vi "Restore Startup Configuration.vi"(8 "error in (no error)":errorcluster, 10 "Startup Configuration File":path=path "C:/Data/Config/start-up.cfg", 11 "Monitor-Pulse in":refnum<class "LabActor.lvclass">) -> (0 "error out":errorcluster, 2 "Startup Configuration":T1={"Load Modules"=[], "External Modules Loaders"=[], "Root Data Folder"=path "C:/Data"}, 3 "Monitor-Pulse out":refnum<class "LabActor.lvclass">)   [LabVIEW 2018, in "LabActor.lvclass"]
uses:
  LabActor.lvclass
  Controllers/Application Controller/Start-up Configuration.ctl
  Controllers/Application Controller/Module Types.ctl
  LabActor.lvclass/LabActor.ctl
  <vilib>/Utility/error.llb/Error Cluster From Error Code.vi
  <vilib>/ErrorRing/Error Ring.xnode
  Controllers/Application Controller/Application Controller.lvclass
  <vilib>/Utility/config.llb/NI_LVConfig.lvlib
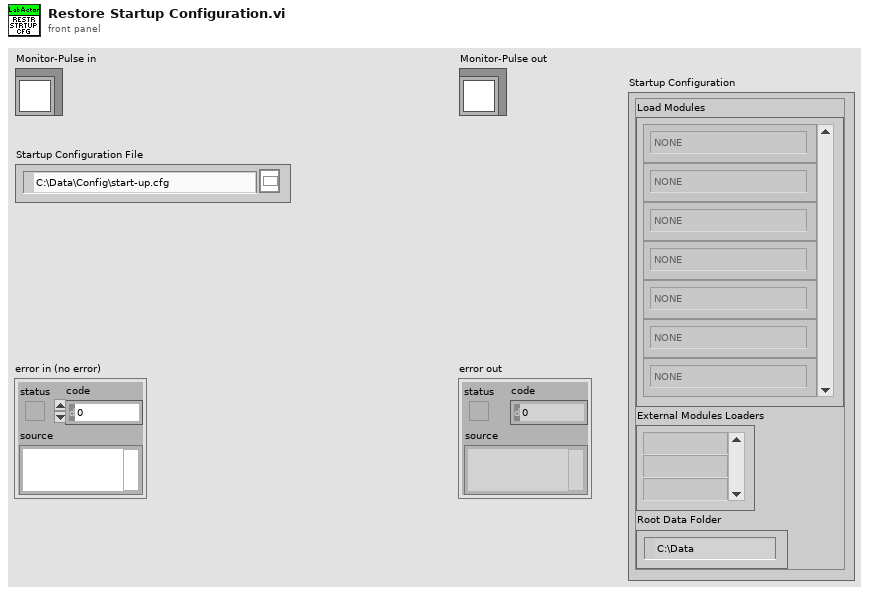
[diagram p1: front panel]
types:
  T1 = typedef "Start-up Configuration.ctl" = cluster{"Load Modules":T2[], "External Modules Loaders":string[], "Root Data Folder":path}
  T2 = typedef "Module Types.ctl" = enum16{"NONE", "NI-DAQmx", "NI-Scope", "Red Pitaya Digitizer", "GaGe", "VISA Device", "Red Pitaya Lockin", "Monitor Controller", "Pulse Controller", "Integrate Pulse", "Lockin Processor", "File converter", "NHMFL Synthesizer", "Micron Hyperion", "Spectrum Recorder", "Resonance Detector", "TCP Communications", "Format Resonances", "Ruby Spectra", "PID Controller"}
  T3 = typedef "NI_LVConfig.lvlib/Config Data RefNum.ctl" = refnum<k1>
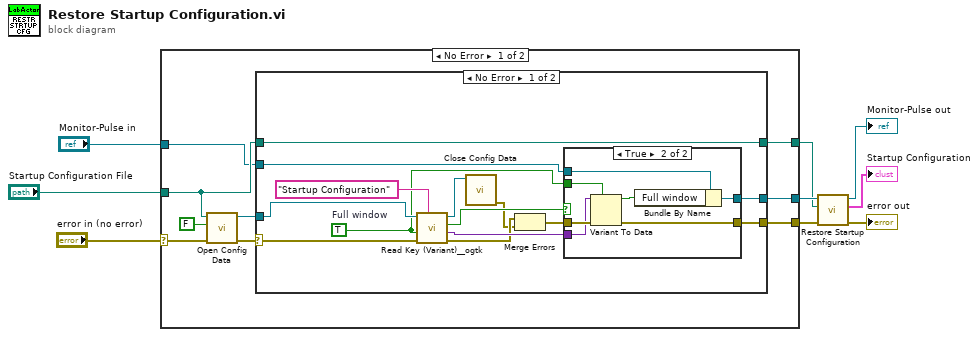
[diagram p0: block diagram]
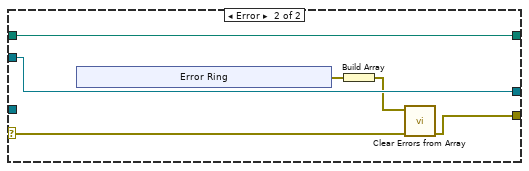
[diagram p3: hidden frame]
diagram:
  n1 = case shown="No Error" "error in (no error)" {
    selector: "error in (no error)" -> [w13 w54]
    tunnel: [w11 w54] -> w2
    tunnel: [w17 w53] -> w3
    tunnel: "Monitor-Pulse in" -> [w12 w53]
    tunnel: "Startup Configuration File" -> [w14 w52]
    tunnel: [w10 w52] -> w1
    frame No Error {
      n2 = call <vilib>:"Open Config Data.vi"("error in (no error)"=w13, "create file if necessary (T)"=FALSE, "configuration file path"=w14) -> ("error out"=w16:errorcluster, "refnum"=w18:T3)  [unwired: 6 in, 1 out]
      n3 = case shown="No Error" w16 {
        selector: w16 -> [w22 w47]
        tunnel: w12 -> [w21 w46]
        tunnel: w18 -> [w31 _]
        tunnel: [w30 w46] -> w17
        tunnel: [w28 w45] -> w11
        tunnel: w14 -> [w20 w42]
        tunnel: [w20 w42] -> w10
        frame No Error {
          w19 = TRUE  # Full window
          n4 = call <userlib>:"Read Key (Variant)__ogtk.vi"("section"="Startup Configuration", "error in (no error)"=w22, "type"=w19, "refnum"=w31) -> ("error out"=w26:errorcluster, "key-value"=w29:variant, "found?"=w27:bool, "refnum out"=w25:T3)  [unwired: 4 in]
          n5 = call <vilib>:"Close Config Data.vi"("refnum"=w25) -> ("error out"=w24:errorcluster)  [unwired: 9 in, 1 out]
          n6 = Merge Errors(w26, w24) -> (w23:errorcluster)
          n7 = case shown="True" w27 {
            tunnel: w21 -> [w34 w41]
            tunnel: [w34 w40] -> w30
            tunnel: w23 -> [w33 w39]
            tunnel: w29 -> [_ w38]
            tunnel: w19 -> [_ w37]
            tunnel: [w33 w35] -> w28
            frame False {
            }
            frame True {
              n8 = Variant To Data(error in=w39, type=w37, Variant=w38) -> (data=w36:bool, error out=w35:errorcluster)
              n9 = Bundle By Name(cluster=w41, "Full window"=w36) -> (w40:refnum<class "LabActor.lvclass">)
            }
          }
        }
        frame Error {
          n10 = xnode "Error Ring"() -> ("error out"=w44:errorcluster)
          n11 = Build Array(w44) -> (w43:errorcluster[])
          n12 = call "Clear Errors from Array.vi"("Error In"=w47, "Errors to clear"=w43) -> ("Error Out"=w45:errorcluster)  [unwired: 8 in, 1 out]
        }
      }
    }
    frame Error {
    }
  }
  n13 = call-parent "Restore Startup Configuration.vi"("error in (no error)"=w2, "Startup Configuration File"=w1, "Monitor-Pulse in"=w3) -> ("error out"=→"error out":errorcluster, "Startup Configuration"=→"Startup Configuration":T1, "Monitor-Pulse out"=→"Monitor-Pulse out":refnum<class "LabActor.lvclass">)  [unwired: 6 in]
